vi "UI.vi"() -> ()   [LabVIEW 2017]
uses:
  <vilib>/Instr/_visa.llb/VISA Configure Serial Port (Instr).vi
  <vilib>/addons/Biomedical/Biosignal Measurements/Biosignal Preprocessing/Biosignal Rate Extractor (Waveform).vi
  <vilib>/addons/Biomedical/NI_BMTK_Measurements.lvlib
panel:
  out "Heart rate":i32
  out "CH2     RPM":dbl
  out "CH1     RPM":dbl
  out "Ch2":waveform(dbl)(graph)
  out "CH1":waveform(dbl)(graph)
  in  "stop":bool
  in  "Arduino Port":refnum<visa-resource-name>
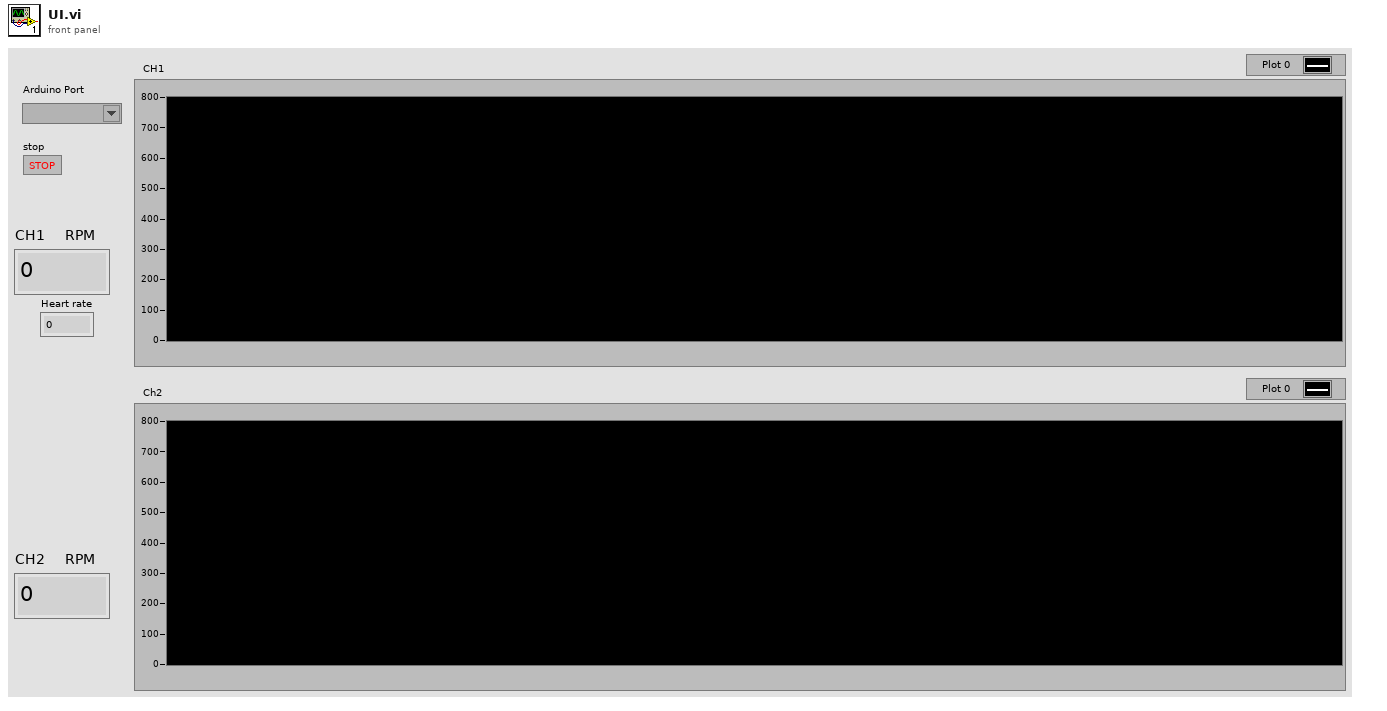
[diagram p1: front panel]
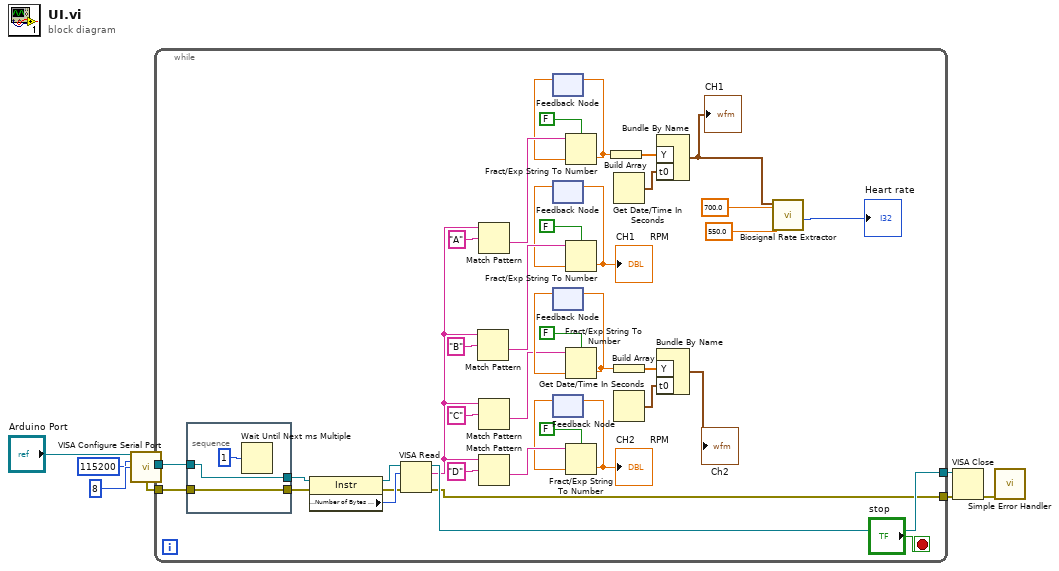
[diagram p0: block diagram]
diagram:
  n1 = call-poly "VISA Configure Serial Port"("VISA resource name"="Arduino Port", "baud rate (9600)"=u32 115200, "data bits (8)"=u16 8) -> ("VISA resource name out"=w5:refnum<visa-resource-name>, "error out"=w4:errorcluster)  [unwired: 11 in]
  n2 = while {
    tunnel: w5 -> [w48]
    tunnel: w4 -> [w46]
    tunnel: [w32] -> w3
    tunnel: [w13] -> w2
    stop <- "stop" stop-if-true
    n3 = stacked-sequence {
      tunnel: w48 -> [w51]
      tunnel: [w51] -> w47
      tunnel: w46 -> [w50]
      tunnel: [w50] -> w45
      frame #0 {
        n4 = Wait Until Next ms Multiple(millisecond multiple=u32 1) -> ()  [unwired: 1 out]
      }
    }
    n5 = property class="Instr"(reference=w47, error in=w45) -> (reference out=w44:refnum<visa-resource-name>, error out=w42:errorcluster, "Serial Settings:Number of Bytes at Serial Port"=w43:u32)
    n6 = VISA Read(VISA resource name=w44, byte count=w43, error in (no error)=w42) -> (VISA resource name out=w32:refnum<visa-resource-name>, read buffer=w22:string, error out=w13:errorcluster)  [unwired: 1 out]
    n7 = Match Pattern(string=w22, regular expression="B") -> (after substring=w37:string)  [unwired: 1 in, 3 out]
    n8 = Match Pattern(string=w22, regular expression="A") -> (after substring=w38:string)  [unwired: 1 in, 3 out]
    n9 = Match Pattern(string=w22, regular expression="C") -> (after substring=w29:string)  [unwired: 1 in, 3 out]
    n10 = Match Pattern(string=w22, regular expression="D") -> (after substring=w25:string)  [unwired: 1 in, 3 out]
    n11 = feedback #1() -> (w34:dbl)  [unwired: 1 in]
    n12 = feedback #2() -> (w33:dbl)  [unwired: 1 in]
    n13 = feedback #3() -> (w31:dbl)  [unwired: 1 in]
    n14 = feedback #4() -> (w24:dbl)  [unwired: 1 in]
    n15 = Fract/Exp String To Number(use system decimal point (T)=FALSE, string=w38, default (0 dbl)=w34) -> (number=w18:dbl)  [unwired: 1 in, 1 out]
    n16 = feedback-in #1(w18) -> ()
    n17 = Fract/Exp String To Number(use system decimal point (T)=FALSE, string=w37, default (0 dbl)=w33) -> (number=w27:dbl)  [unwired: 1 in, 1 out]
    "CH1     RPM" <- w27
    n18 = feedback-in #2(w27) -> ()
    n19 = Fract/Exp String To Number(use system decimal point (T)=FALSE, string=w29, default (0 dbl)=w31) -> (number=w17:dbl)  [unwired: 1 in, 1 out]
    n20 = feedback-in #3(w17) -> ()
    n21 = Fract/Exp String To Number(use system decimal point (T)=FALSE, string=w25, default (0 dbl)=w24) -> (number=w23:dbl)  [unwired: 1 in, 1 out]
    "CH2     RPM" <- w23
    n22 = feedback-in #4(w23) -> ()
    n23 = Build Array(w18) -> (w19:dbl[])
    n24 = Get Date/Time In Seconds() -> (seconds since 1Jan1904=w14:timestamp)
    n25 = Build Array(w17) -> (w16:dbl[])
    n26 = Get Date/Time In Seconds() -> (seconds since 1Jan1904=w15:timestamp)
    n27 = Bundle By Name("Y"=w19, "t0"=w14) -> (w12:waveform(dbl))  [unwired: 1 in]
    "CH1" <- w12
    n28 = Bundle By Name("Y"=w16, "t0"=w15) -> (→"Ch2":waveform(dbl))  [unwired: 1 in]
    n29 = call-poly <vilib>:"Biosignal Rate Extractor.vi"("low threshold"=550.0, "high threshold"=700.0, "biosignal"=w12) -> ("number of cycles per minuets"=→"Heart rate":i32)  [unwired: 5 in, 3 out]
  }
  n30 = VISA Close(VISA resource name=w3, error in (no error)=w2) -> (error out=w1:errorcluster)
  n31 = call <vilib>:"Simple Error Handler.vi"("error in (no error)"=w1) -> ()  [unwired: 4 in, 5 out]
